vi "LoopselFFCont.VI"() -> ()   [LabVIEW 2015]
uses:
  <vilib>/Analysis/NI_AALBase.lvlib
panel:
  in  "EC in 10ns":u32
  out "tRMS":dbl=8.272957184592048 format="%0#.1f"
  out "mean":dbl=3064.5285285285286 format="%#_4f"
  in  "Pixel":u16=100
  in  "alloc mem":bool
  out "FREE \nRAM MB":u64=14063
  out "BUILT-IN\nRAM MB":u64=16662
  out "SEC":dbl=0.04
  out "MB RAM":u64=2
  in  "pos slope":u8=1
  in  "both slopes":u8
  in  "DAT in 10ns":u32
  out "FIFO overflow":bool
  in  "extTrig 0/1":u8
  in  "stop all":bool
  in  "start new block":bool
  in  "Slide":u32(slide)=387 scale=1.0..1000.0
  in  "frequency[Hz]":u32
  in  "no.of samples (nos)":u32=1000
  in  "exposuretime[ms]":dbl=0.04 format="%.3f"
  out "Signalverlaufgraph":u16[](graph)=[3058, 3058, 3058, 3058, 0, 1, 0, 386, 3066, 3054, 3068, 3076, 3068, 3074, 3074, 3080, 3068, 3064, 3076, 3064, 3074, 3058, 3064, 3082, 3058, 3084, 3070, 3074, 3084, 3066, 3070, 3070, 3062, 3072, 3074, 3074, 3070, 3066, 3068, 3068, 3082, 3064, 3068, 3070, 3056, 3058, 3066, 3076, 3066, 3060, 3072, 3072, 3076, 3082, 3062, 3062, 3072, 3066, 3054, 3070, 3054, 3074, 3056, 3076, 3068, 3058, 3068, 3080, 3070, 3058, 3052, 3062, 3064, 3060, 3060, 3068, 3072, 3072, 3060, 3054, 3058, 3060, 3064, 3058, 3058, 3062, 3066, 3064, 3042, 3062, 3066, 3060, 3062, 3052, 3062, 3058, 3056, 3052, 3060, 3062, 3068, 3048, 3056, 3074, 3070, 3054, 3062, 3064, 3052, 3062, 3064, 3074, 3068, 3064, 3058, 3060, 3074, 3062, 3064, 3062, 3052, 3052, 3054, 3058, 3058, 3054, 3052, 3064, 3064, 3062, 3064, 3056, 3064, 3050, 3048, 3048, 3050, 3036, 3044, 3056, 3032, 3052, 3048, 3054, 3034, 3040, 3050, 3044, 3042, 3028, 3036, 3056, 3046, 3050, 3060, 3052, 3048, 3036, 3044, 3054, 3052, 3048, 3042, 3038, 3040, 3044, 3052, 3036, 3050, 3048, 3046, 3052, 3044, 3042, 3044, 3052, 3034, 3040, 3048, 3044, 3052, 3044, 3046, 3034, 3030, 3032, 3024, 3032, 3026, 3046, 3036, 3052, 3046, 3030, 3050, 3042, 3046, 3038, 3026, 3050, 3040, 3038, 3038, 3034, 3044, 3052, 3052, 3024, 3038, 3040, 3040, 3032, 3034, 3042, 3042, 3028, 3030, 3044, 3046, 3040, 3044, 3026, 3028, 3036, 3014, 3036, 3036, 3036, 3036, 3016, 3032, 3040, 3038, 3028, 3042, 3026, 3038, 3030, 3050, 3040, 3044, 3036, 3036, 3032, 3044, 3038, 3046, 3032, 3024, 3030, 3030, 3042, 3024, 3024, 3034, 3044, 3044, 3036, 3034, 3026, 3026, 3032, 3022, 3022, 2990, 2976, 2986, 2992, 2980, 2980, 3000, 2996, 2990, 2980, 2982, 2988, 2996, 2980, 2986, 3004, 2988, 3004, 2994, 2994, 3002, 2998, 2990, 2996, 2992, 2986, 2996, 2992, 2990, 2990, 2994, 2990, 2994, 2990, 2984, 2990, 2984, 2980, 2984, 3002, 2982, 2988, 2988, 2988, 2984, 2990, 2984, 2974, 2998, 2982, 2968, 2976, 2976, 2988, 2982, 3000, 2996, 2980, 2986, 2996, 2986, 2982, 2962, 2996, 2992, 2976, 2988, 2986, 2974, 2992, 2978, 2976, 2980, 2984, 2986, 2978, 2980, 2976, 2984, 2974, 2970, 2982, 2984, 2990, 2980, 2976, 2970, 2970, 2974, 2970, 2988, 2978, 2984, 2970, 2978, 2994, 2990, 2976, 2968, 2968, 2980, 2972, 2996, 2986, 2978, 2996, 2976, 2978, 2990, 2976, 2982, 2982, 2972, 2982, 2974, 2972, 2966, 2974, 2968, 2986, 2984, 2984, 2970, 2976, 2978, 2964, 2968, 2968, 2986, 2972, 2988, 2990, 2982, 2988, 2994, 2992, 2984, 2978, 2984, 2988, 2990, 2982, 2996, 3008, 2988, 2998, 2990, 2990, 2988, 2990, 2982, 2982, 2990, 2980, 2990, 2990, 2996, 2990, 2986, 2994, 2994, 2980, 2990, 2990, 2978, 2978, 2982, 2994, 2978, 2988, 2992, 2994, 2986, 2990, 2978, 2970, 2992, 2988, 2966, 2970, 2980, 2986, 2984, 2982, 2986, 2976, 2992, 2984, 2998, 2986, 2974, 2986, 2982, 2970, 2982, 2990, 2980, 2988, 2990, 2974, 2980, 2976, 2990, 2976, 2976, 2982, 2978, 2978, 2968, 2976, 2994, 2980, 2994, 2966, 2972, 2964, 2964, 2970, 2976, 2982, 2976, 2958, 2974, 2986, 2986, 2978, 2990, 2982, 2978, 2970, 2992, 2980, 2972, 2980, 2982, 2978, 2990, 2982, 2976, 2978, 2978, 2972, 2974, 2976, 2976, 2972, 2974, 2978, 2982, 2982, 2988, 2964, 2986, 2974, 2958, 2958, 2988, 2980, 2984, 2990, 2984, 2988, 2994, 2998, 3002, 2988, 2986, 2992, 2998, 2988, 2994, 3004, 2992, 3006, 2994, 3002, 3004, 3002, 2998, 2988, 2992, 2996, 3010, 2988, 2984, 3002, 2990, 2990, 2998, 2986, 2992, 2996, 2980, 2988, 2986, 2994, 2986, 2996, 3002, 2994, 2996, 2990, 2992, 2980, 2998, 2984, 2974, 2974, 2982, 2992, 2992, 2998, 2990, 2984, 3002, 2994, 3000, 2982, 2970, 2996, 2996, 2982, 2992, 2988, 2992, 2994, 2980, 2982, 2988, 2986, 2986, 2996, 2996, 2998, 2988, 2974, 2968, 2982, 2990, 2982, 2984, 2976, 2990, 2978, 2970, 2982, 2984, 2990, 2984, 2970, 2972, 2996, 2994, 2982, 2982, 2994, 2982, 2976, 2990, 2994, 2990, 2990, 2984, 2980, 2990, 2978, 2986, 2984, 2980, 2992, 2982, 2982, 2974, 2982, 2976, 2986, 2994, 2990, 2990, 2980, 2982, 2976, 2974, 2974, 3016, 3010, 3020, 3018, 3000, 3022, 3022, 3024, 3010, 3012, 3014, 3014, 3008, 3006, 3020, 3032, 3018, 3022, 3014, 3026, 3018, 3014, 3026, 3010, 3014, 3010, 3018, 3008, 3016, 3018, 3008, 3010, 3016, 3008, 3020, 3020, 3002, 3004, 3006, 3016, 3006, 3012, 3020, 3016, 3018, 3016, 3008, 2992, 3014, 3018, 3002, 3010, 3008, 3008, 3008, 3018, 3012, 3012, 3016, 3010, 3016, 3014, 2992, 3026, 3012, 3014, 3014, 3008, 3004, 3020, 3010, 3002, 3006, 3010, 3014, 3012, 3014, 3020, 3008, 3004, 3000, 3004, 3008, 3006, 3016, 3002, 3002, 2994, 2984, 2996, 3000, 3006, 3018, 2994, 3000, 3010, 3016, 2998, 3006, 3006, 3006, 2994, 3018, 3012, 3022, 3000, 3012, 3004, 3020, 3012, 3020, 3010, 3002, 3002, 3016, 3002, 2994, 2996, 2994, 3014, 3010, 3006, 3012, 3006, 3002, 3002, 2988, 2988, 3018, 3008, 3008, 3020, 3010, 3006, 3018, 3020, 3010, 3002, 3002, 3008, 3006, 2998, 3012, 3024, 3000, 3020, 3014, 3004, 3002, 3006, 3010, 2994, 3014, 3018, 3024, 2996, 3006, 3008, 3008, 3004, 3012, 3004, 3012, 3018, 2998, 3012, 3010, 3016, 3006, 3008, 3004, 3010, 3008, 3010, 2996, 2992, 3008, 3006, 2990, 2986, 2990, 3006, 2996, 3014, 3006, 2998, 3018, 3020, 3006, 2992, 2990, 3004, 3008, 3002, 2996, 3006, 3006, 3012, 2996, 2994, 3002, 2998, 3008, 3002, 2994, 3004, 3008, 2986, 2984, 2992, 3016, 3002, 3006, 2998, 3002, 2992, 2988, 2986, 2988, 3006, 2998, 2982, 2988, 3004, 3006, 2992, 3000, 3008, 2996, 2994, 3004, 3004, 3002, 3010, 2996, 2996, 3014, 2994, 2998, 2996, 2998, 2998, 2998, 2992, 2990, 2998, 3004, 3010, 2998, 3004, 2998, 3000, 3000, 2988, 2982, 2982, 3052, 3046, 3036, 3042, 3036, 3046, 3054, 3058, 3046, 3042, 3050, 3040, 3038, 3032, 3042, 3060, 3052, 3058, 3044, 3054, 3048, 3040, 3038, 3040, 3044, 3040, 3044, 3040, 3036, 3044, 3050, 3054, 3040, 3038, 3050, 3050, 3036, 3032, 3044, 3054, 3032, 3046, 3050, 3054, 3042, 3050, 3036, 3024, 3044, 3044, 3028, 3036, 3028, 3042, 3040, 3054, 3040, 3036, 3046, 3054, 3040, 3030, 3016, 3046, 3040, 3030, 3042, 3044, 3048, 3054, 3036, 3036, 3036, 3048, 3036, 3032, 3032, 3042, 3046, 3028, 3022, 3030, 3048, 3032, 3048, 3018, 3024, 3022, 3018, 3030, 3042, 3030, 3028, 3020, 3024, 3044, 3040, 3030, 3030, 3040, 3036, 3022, 3056, 3038, 3036, 3038, 3036, 3030, 3044, 3034, 3038, 3026, 3032, 3022, 3030, 3036, 3022, 3038, 3028, 3040, 3032, 3032, 3034, 3018, 3040, 3024, 3030, 3030, 3058, 3052, 3062, 3054, 3056, 3062, 3054, 3046, 3070, 3064, 3054, 3058, 3054, 3058, 3058, 3058, 3052, 3060, 3042, 3048, 3052, 3052, 3048, 3056, 3044, 3068, 3058, 3050, 3058, 3050, 3058, 3058, 3066, 3062, 3062, 3056, 3058, 3070, 3052, 3064, 3066, 3060, 3048, 3058, 3068, 3046, 3050, 3064, 3052, 3070, 3052, 3064, 3056, 3056, 3056, 3056]
  # "Start with run"
  # "Abort with ESC"
  # "1x"
  # "repeat"
  # "exit here"
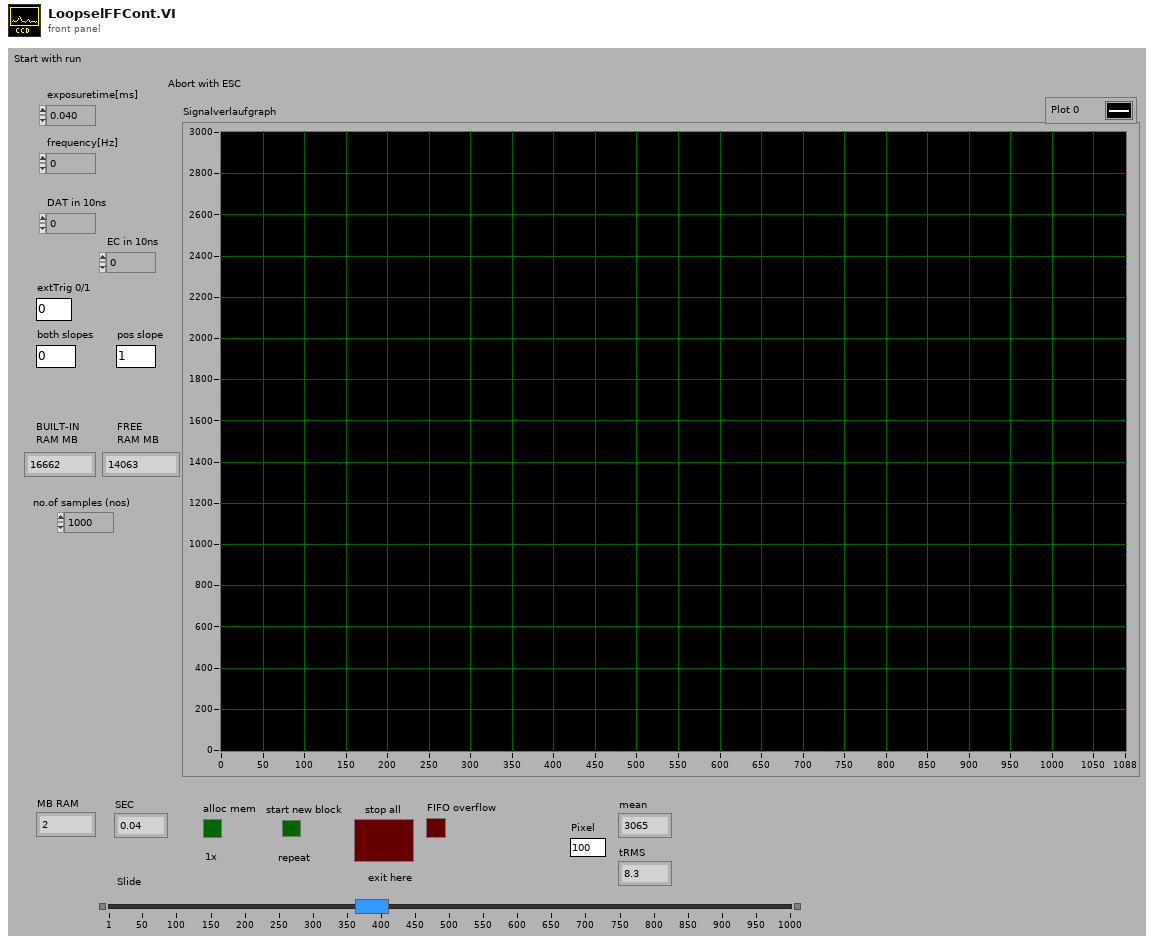
[diagram p1: front panel]
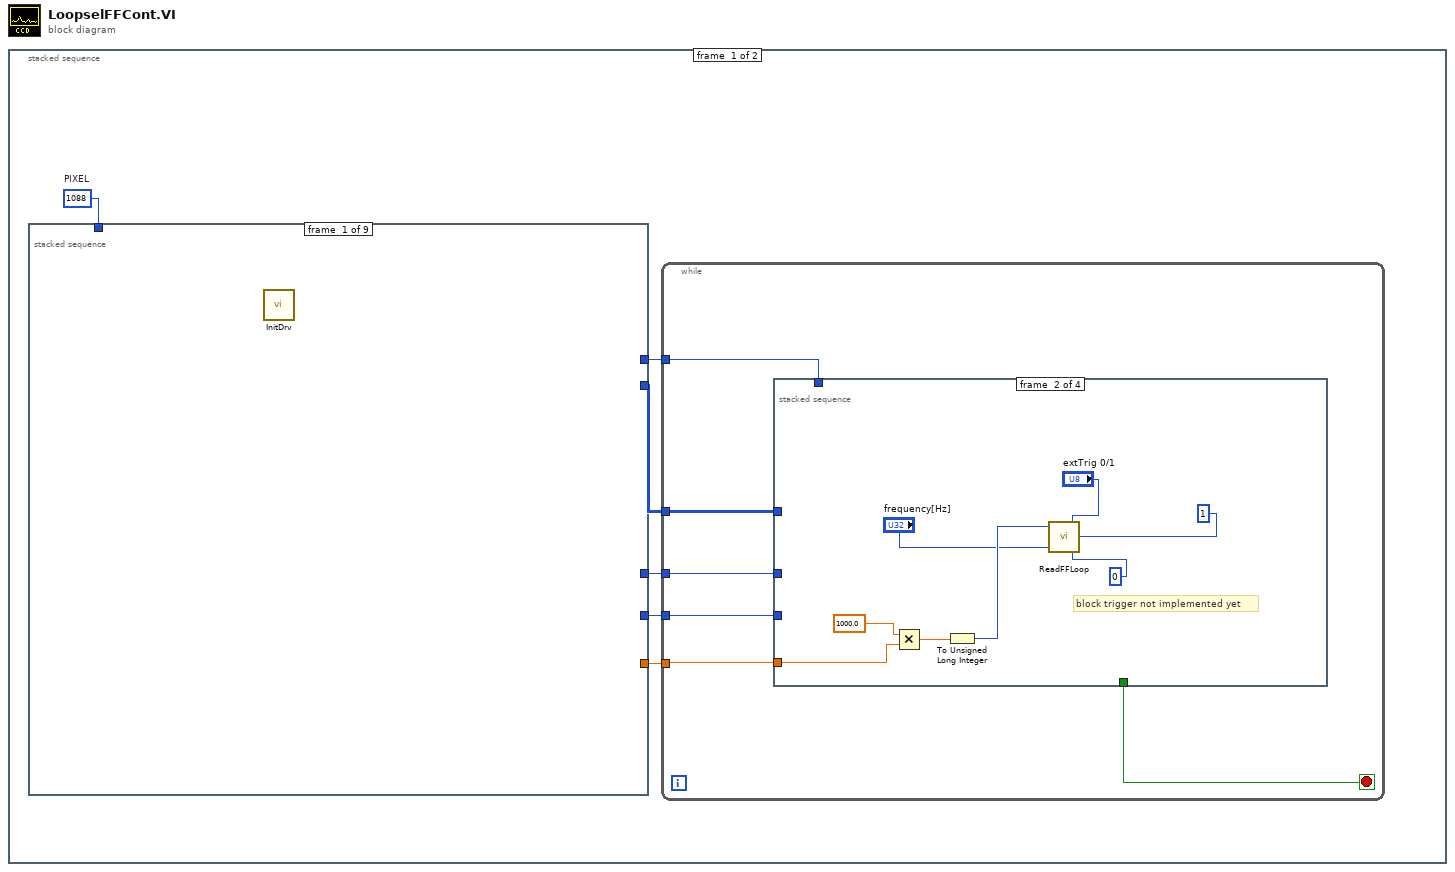
[diagram p0: block diagram]
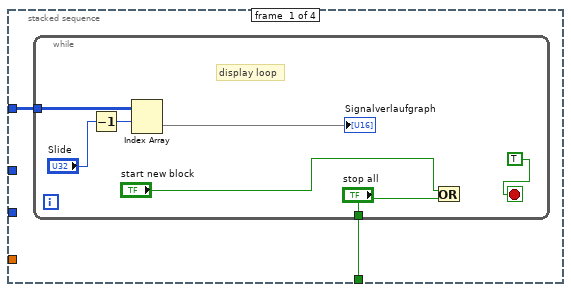
[diagram p2: hidden frame]
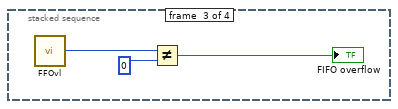
[diagram p3: hidden frame]
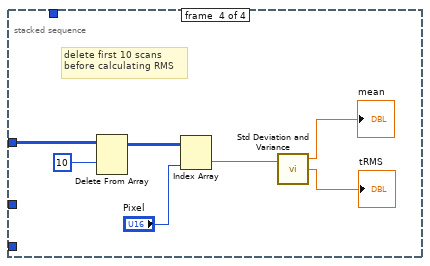
[diagram p4: hidden frame]
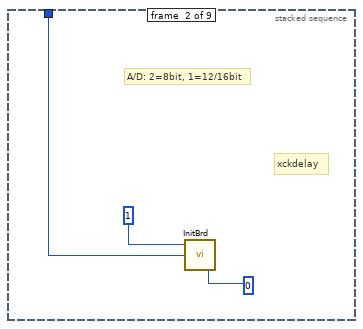
[diagram p5: hidden frame]
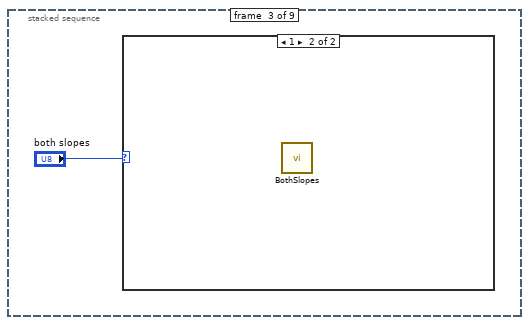
[diagram p6: hidden frame]
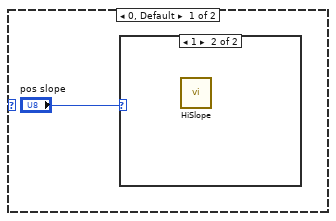
[diagram p7: hidden frame]
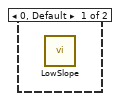
[diagram p8: hidden frame]
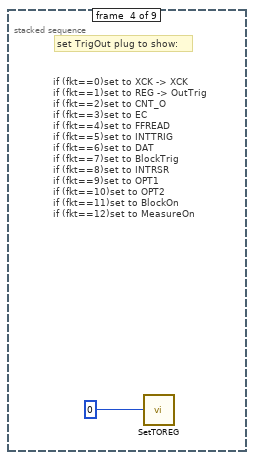
[diagram p9: hidden frame]
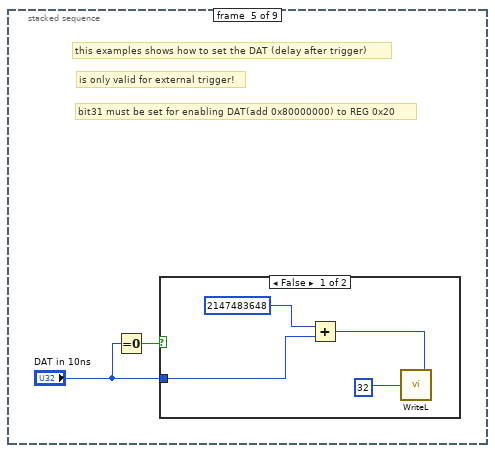
[diagram p10: hidden frame]
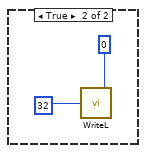
[diagram p11: hidden frame]
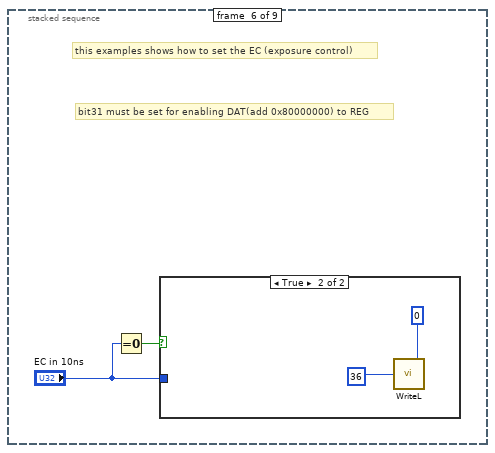
[diagram p12: hidden frame]
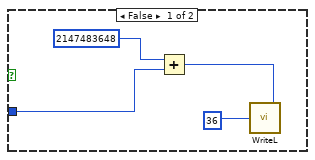
[diagram p13: hidden frame]
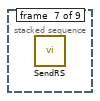
[diagram p14: hidden frame]
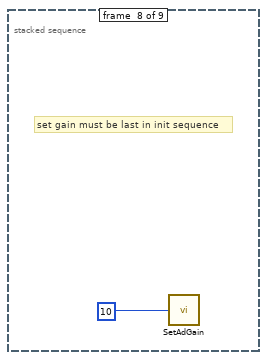
[diagram p15: hidden frame]
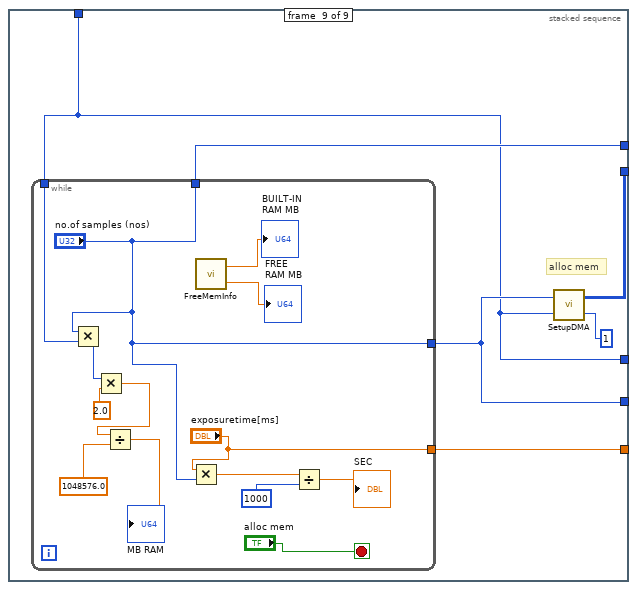
[diagram p16: hidden frame]
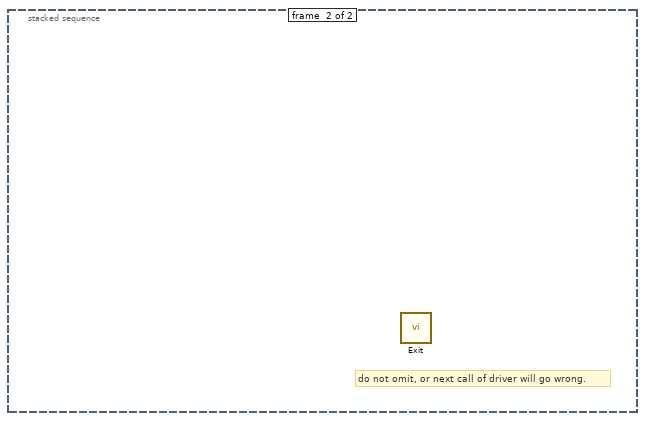
[diagram p17: hidden frame]
diagram:
  n1 = stacked-sequence {
    frame #0 {
      w3 = u32 1088  # PIXEL
      n2 = stacked-sequence {
        tunnel: [_ _ _ _ _ _ _ _ w68] -> w6
        tunnel: [_ _ _ _ _ _ _ _ w65] -> w5
        tunnel: [_ _ _ _ _ _ _ _ w66] -> w4
        tunnel: w3 -> [_ w40 _ _ _ _ _ _ w63]
        tunnel: [_ _ _ _ _ _ _ _ w64] -> w2
        tunnel: [_ _ _ _ _ _ _ _ w63] -> w1
        frame #0 {
          n3 = call "InitDrv.vi"() -> ()  [unwired: 1 in, 1 out]
        }
        frame #1 {
          # "xckdelay"
          # "A/D: 2=8bit, 1=12/16bit"
          n4 = call "InitBrd.vi"("xckdly"=u32 0, "pixel"=w40, "flag816"=u32 1) -> ()  [unwired: 3 in]
        }
        frame #2 {
          n5 = case shown="1" "both slopes" {
            frame 0, Default {
              n6 = case shown="1" "pos slope" {
                frame 0, Default {
                  n7 = call "LowSlope.vi"() -> ()  [unwired: 1 in]
                }
                frame 1 {
                  n8 = call "HiSlope.vi"() -> ()  [unwired: 1 in]
                }
              }
            }
            frame 1 {
              n9 = call "BothSlopes.vi"() -> ()  [unwired: 1 in]
            }
          }
        }
        frame #3 {
          # "if (fkt==0)set to XCK -> XCK\nif (fkt==1)set to REG -> OutTrig\nif (fkt==2)set to CNT_O\nif (fkt==3)set to EC\nif (fkt==4)set to FFREAD\nif (fkt==5)set to INTTRIG\nif (fkt==6)set to DAT\nif (fkt==7)set to BlockTrig\nif (fkt==8)set to INTRSR\nif (fkt==9)set to OPT1\nif (fkt==10)set to OPT2\nif (fkt==11)set to BlockOn\nif (fkt==12)set to MeasureOn"
          # "set TrigOut plug to show:"
          n10 = call "SetTOREG.vi"("fkt"=u8 0) -> ()
        }
        frame #4 {
          # "bit31 must be set for enabling DAT(add 0x80000000) to REG 0x20"
          # "is only valid for external trigger!"
          # "this examples shows how to set the DAT (delay after trigger)"
          n11 = Equal To 0?(x="DAT in 10ns") -> (x = 0?=w47:bool)
          n12 = case shown="False" w47 {
            tunnel: "DAT in 10ns" -> [w48 _]
            frame False {
              n13 = Add(x=u32 2147483648, y=w48) -> (x+y=w51:u32)
              n14 = call "WriteL.vi"("val"=w51, "offset"=u32 32) -> ()
            }
            frame True {
              n15 = call "WriteL.vi"("val"=0, "offset"=u32 32) -> ()
            }
          }
        }
        frame #5 {
          # "bit31 must be set for enabling DAT(add 0x80000000) to REG"
          # "this examples shows how to set the EC (exposure control)"
          n16 = Equal To 0?(x="EC in 10ns") -> (x = 0?=w55:bool)
          n17 = case shown="True" w55 {
            tunnel: "EC in 10ns" -> [w56 _]
            frame False {
              n18 = Add(x=u32 2147483648, y=w56) -> (x+y=w59:u32)
              n19 = call "WriteL.vi"("val"=w59, "offset"=u32 36) -> ()
            }
            frame True {
              n20 = call "WriteL.vi"("val"=0, "offset"=u32 36) -> ()
            }
          }
        }
        frame #6 {
          n21 = call "SendRS.vi"() -> ()  [unwired: 1 in]
        }
        frame #7 {
          # "set gain must be last in init sequence"
          n22 = call "SetAdGain.vi"("gain"=u8 10) -> ()  [unwired: 1 in]
        }
        frame #8 {
          # "alloc mem"
          n23 = while {
            tunnel: w63 -> [w78]
            tunnel: ["exposuretime[ms]"] -> w66
            tunnel: ["no.of samples (nos)"] -> w65
            tunnel: ["no.of samples (nos)"] -> w64
            stop <- "alloc mem" stop-if-true
            n24 = Multiply(x="no.of samples (nos)", y=w78) -> (x*y=w79:u32)
            n25 = Multiply(x=w79, y=2.0) -> (x*y=w80:dbl)
            n26 = Divide(x=w80, y=1048576.0) -> (x/y=→"MB RAM":dbl)
            n27 = Multiply(x="exposuretime[ms]", y="no.of samples (nos)") -> (x*y=w75:dbl)
            n28 = call "FreeMemInfo.vi"() -> ("PhysicalSpace"=→"BUILT-IN\nRAM MB":dbl, "PhysicalFreeSpace"=→"FREE \nRAM MB":dbl)  [unwired: 1 in]
            n29 = Divide(x=w75, y=1000) -> (x/y=→"SEC":dbl)
          }
          n30 = call "SetupDMA.vi"("blocks"=1, "pixel"=w63, "nos"=w65) -> ("Data Values"=w68:u16[][])
        }
      }
      n31 = while {
        tunnel: w6 -> [w9]
        tunnel: w5 -> [w12]
        tunnel: w4 -> [w11]
        tunnel: w2 -> [w8]
        tunnel: w1 -> [w7]
        stop <- w10 stop-if-true
        n32 = stacked-sequence {
          tunnel: w9 -> [w14 _ _ w36]
          tunnel: w12 -> [_ _ _ _]
          tunnel: w11 -> [_ w23 _ _]
          tunnel: [w13 _ _ _] -> w10
          tunnel: w8 -> [_ _ _ _]
          tunnel: w7 -> [_ _ _ _]
          frame #0 {
            n33 = while {
              tunnel: w14 -> [w19]
              tunnel: ["stop all"] -> w13
              stop <- TRUE stop-if-true
              # "display loop"
              n34 = Decrement(x="Slide") -> (x-1=w21:u32)
              n35 = Index Array(array=w19, index (row)=w21) -> (element=→"Signalverlaufgraph":u16[])  [unwired: 1 in]
              n36 = Or(x="start new block", y="stop all") -> ()  [unwired: 1 out]
            }
          }
          frame #1 {
            # "block trigger not implemented yet"
            n37 = Multiply(x=1000.0, y=w23) -> (x*y=w24:dbl)
            n38 = To Unsigned Long Integer(number=w24) -> (unsigned 32bit integer=w29:u32)
            n39 = call "ReadFFLoop.vi"("blocktrigger"=u8 0, "btrig_ch"=u8 1, "ExtTrig"="extTrig 0/1", "cam_sel"="frequency[Hz]", "exptus"=w29) -> ()  [unwired: 1 in]
          }
          frame #2 {
            n40 = call "FFOvl.vi"() -> ("FFOvl"=w31:u8)  [unwired: 1 in]
            n41 = Not Equal?(x=w31, y=0) -> (x != y?=→"FIFO overflow":bool)
          }
          frame #3 {
            # "delete first 10 scans\nbefore calculating RMS"
            n42 = Delete From Array(array=w36, index (row)=10) -> (array with subset deleted=w35:u16[][])  [unwired: 2 in, 1 out]
            n43 = Index Array(array=w35, index (col)="Pixel") -> (element=w33:u16[])  [unwired: 1 in]
            n44 = call <vilib>:"Std Deviation and Variance.vi"("X"=w33) -> ("mean"=→"mean":dbl, "standard deviation"=→"tRMS":dbl)  [unwired: 1 in, 1 out]
          }
        }
      }
    }
    frame #1 {
      # "do not omit, or next call of driver will go wrong."
      n45 = call "Exit.vi"() -> ()  [unwired: 1 in]
    }
  }
